vi "XIPIN_AXI_UART16550_2_0.vi"   [LabVIEW 2017]
doc: "The AXI Universal Asynchronous Receiver Transmitter (UART) 16550 connects to the AMBA?(Advance Microcontroller Bus Architecture) AXI (Advanced eXtensible Interface) and provides the controller interface for asynchronous serial data transfer\n------------------------------------\n<b>Need License</b> : No\n<b>Interface</b> : AXI4"
uses:
  <vilib>/rvi/XilinxIP/XIPIN_XNode/niFpgaXIPIN.xnode
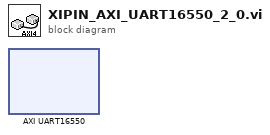
[diagram p0: block diagram]
diagram:
  n1 = xnode ("AXI UART16550")() -> ()
